vi "USB - Asynchronous Read of One JSON Message.vi"(8 "error in":errorcluster, 11 "VISA resource name in":refnum<visa-resource-name>) -> (0 "error out":errorcluster, 2 "Received JSON Message":string, 3 "VISA resource name out":refnum<visa-resource-name>)   [LabVIEW 2021]
doc: "Receive a JSON messsage through USB/Serial"
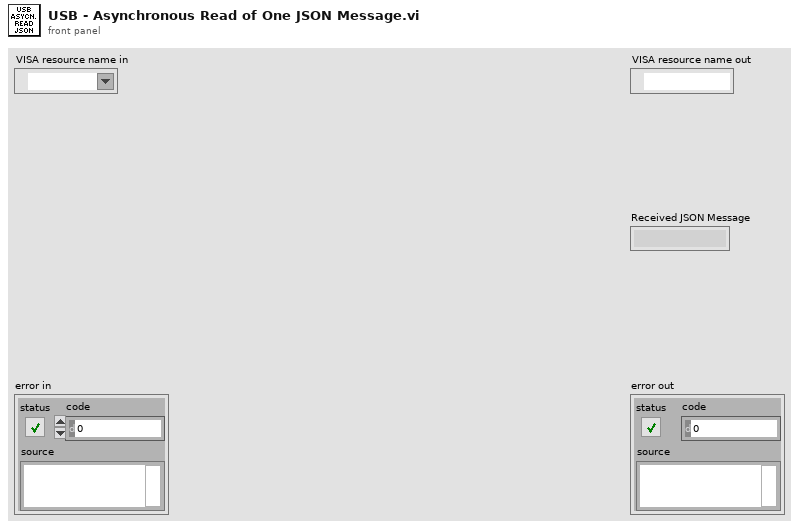
[diagram p1: front panel]
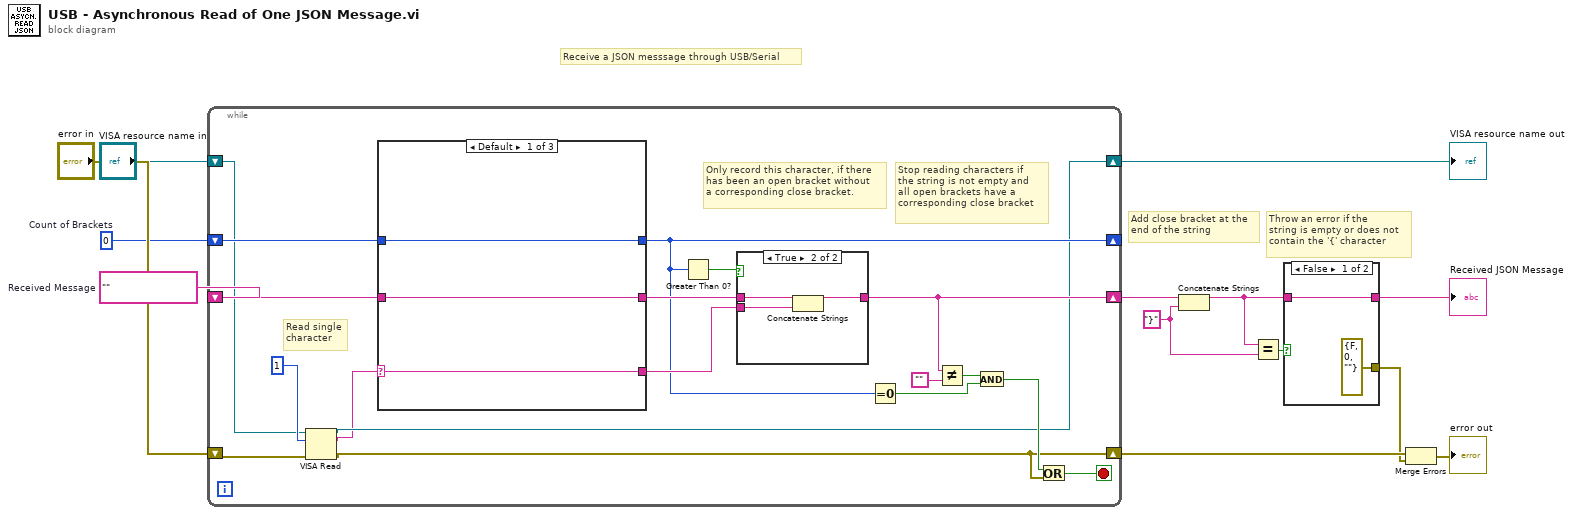
[diagram p0: block diagram]
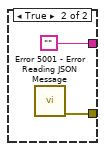
[diagram p2: hidden frame]
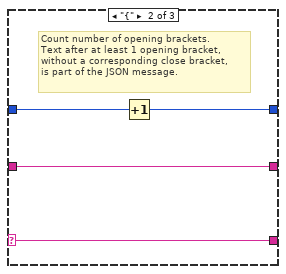
[diagram p4: hidden frame]
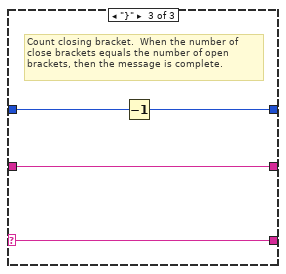
[diagram p5: hidden frame]
diagram:
  w9 = "}" ("string")
  w11 = 0  # Count of Brackets
  w13 = ""  # Received Message
  # "Throw an error if the\nstring is empty or does not\ncontain the '{' character"
  # "Add close bracket at the\nend of the string"
  # "Receive a JSON messsage through USB/Serial"
  n1 = while {
    shift-right: [w18] -> w6
    shift-left: "error in" -> [w19]
    shift-right: [w15] -> w1
    shift-left: "VISA resource name in" -> [w16]
    shift-right: [w24] -> w10
    shift-left: w13 -> [w27]
    shift-right: [w23] -> _
    shift-left: w11 -> [w30]
    stop <- w31 stop-if-true
    # "Stop reading characters if\nthe string is not empty and\nall open brackets have a \ncorresponding close bracket"
    # "Only record this character, if there\nhas been an open bracket without\na corresponding close bracket."
    # "Read single\ncharacter"
    n2 = VISA Read(VISA resource name=w16, byte count=1 ("bytes to read"), error in (no error)=w19) -> (VISA resource name out=w15:refnum<visa-resource-name>, read buffer=w14:string, error out=w18:errorcluster)  [unwired: 1 out]
    n3 = case shown="Default" w14 {
      selector: w14 -> [w36 w40 w43]
      tunnel: w30 -> [w38 w42 w46]
      tunnel: [w38 w41 w45] -> w23
      tunnel: [w36 w40 w43] -> w28
      tunnel: w27 -> [w37 w39 w44]
      tunnel: [w37 w39 w44] -> w26
      frame Default {
      }
      frame "{" {
        # "Count number of opening brackets.  \nText after at least 1 opening bracket, \nwithout a corresponding close bracket, \nis part of the JSON message."
        n4 = Increment(x=w42) -> (x+1=w41:i32)
      }
      frame "}" {
        # "Count closing bracket.  When the number of\nclose brackets equals the number of open \nbrackets, then the message is complete."
        n5 = Decrement(x=w46) -> (x-1=w45:i32)
      }
    }
    n6 = Greater Than 0?(x=w23) -> (x > 0?=w29:bool)
    n7 = case shown="True" w29 {
      tunnel: [w32 w35] -> w24
      tunnel: w28 -> [_ w34]
      tunnel: w26 -> [w32 w33]
      frame False {
      }
      frame True {
        n8 = Concatenate Strings(w33, w34) -> (w35:string)
      }
    }
    n9 = Equal To 0?(x=w23) -> (x = 0?=w21:bool)
    n10 = Not Equal?(x=w24, y="") -> (x != y?=w22:bool)
    n11 = And(x=w22, y=w21) -> (x .and. y?=w20:bool)
    n12 = Or(x=w20, y=w18) -> (x .or. y?=w31:bool)
  }
  "VISA resource name out" <- w1
  n13 = Concatenate Strings(w10, w9) -> (w3:string)
  n14 = Equal?(x=w3, y=w9) -> (x = y?=w7:bool)
  n15 = case shown="False" w7 {
    tunnel: [errorcluster {"status"=FALSE, "code"=0, "source"=""} ("error out") w50] -> w5
    tunnel: [w47 ""] -> w4
    tunnel: w3 -> [w47 _]
    frame False {
    }
    frame True {
      n16 = call "Error 5001 - Error Reading JSON Message.vi"() -> ("error out"=w50:errorcluster)  [unwired: 11 in]
    }
  }
  "Received JSON Message" <- w4
  n17 = Merge Errors(w6, w5) -> (→"error out":errorcluster)
